vi "browse for tdms data file for report.vi"   [LabVIEW 2025]
uses:
  Libraries/Settings Editor/Settings Editor.lvlib
types:
  T1 = typedef "Settings Editor.lvlib/Update Application Settings (Reply Payload)--cluster.ctl" = cluster{"Settings":T2, "error":errorcluster}
  T2 = typedef "Settings Editor.lvlib/Settings--cluster.ctl" = cluster{"Log File Base Path":path, "Meta Data":T3, "DAQ Settings":cluster{"physical channel":string, "minimum value":dbl, "maximum value":dbl, "number of samples":i32, "rate":dbl, "custom scale name":string}, "Report Save Folder":path}
  T3 = typedef "Settings Editor.lvlib/Test Meta Data.ctl" = cluster{"Operator":string, "Job Number":string, "Part Number":string}
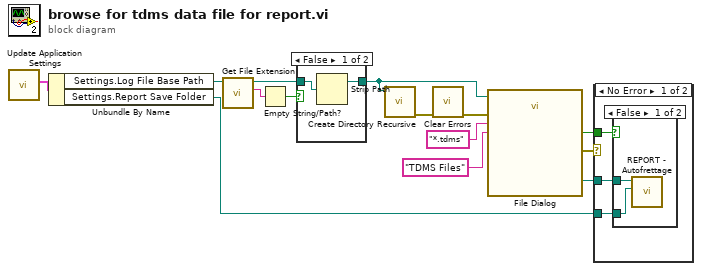
[diagram p0: block diagram]
diagram:
  n1 = call "Update Application Settings.vi"() -> ("Reply Payload"=w8:T1)  [unwired: 9 in, 2 out]
  n2 = Unbundle By Name(w8) -> ("Settings.Log File Base Path"=w7:path, "Settings.Report Save Folder"=w1:path)
  n3 = call <vilib>:"Get File Extension.vi"("file"=w7) -> ("lowercase file extension"=w6:string, "dup file"=w3:path)  [unwired: 6 in, 3 out]
  n4 = Empty String/Path?(string/path=w6) -> (empty?=w5:bool)
  n5 = case shown="False" w5 {
    tunnel: [w15 w17] -> w4
    tunnel: w3 -> [w16 w17]
    frame False {
      n6 = Strip Path(path=w16) -> (stripped path=w15:path)  [unwired: 1 out]
    }
    frame True {
    }
  }
  n7 = call <vilib>:"Create Directory Recursive.vi"("directory"=w4) -> ("error out"=w12:errorcluster)  [unwired: 4 in, 2 out]
  n8 = call <vilib>:"Clear Errors.vi"("error in (no error)"=w12) -> ("error out"=w11:errorcluster)  [unwired: 5 in, 1 out]
  n9 = call "File Dialog"("start path"=w4, "error in"=w11, "pattern (all files)"="*.tdms", "pattern label"="TDMS Files") -> ("selected path"=w14:path, "cancelled"=w13:bool, "error out"=w2:errorcluster)  [unwired: 8 in, 1 out]
  n10 = case shown="No Error" w2 {
    tunnel: w14 -> [w20 _]
    tunnel: w13 -> [w19 _]
    tunnel: w1 -> [w18 _]
    frame No Error {
      n11 = case shown="False" w19 {
        tunnel: w20 -> [w22 _]
        tunnel: w18 -> [w21 _]
        frame False {
          n12 = call "REPORT - Autofrettage.vi"("Report Save Path"=w21, "TDMS file path"=w22) -> ()  [unwired: 10 in]
        }
        frame True {
        }
      }
    }
    frame Error {
    }
  }
